vi "WordWrapping.vi"(1 "FormattedMultiLineStringIn":string="123<B>ABCD</B>456\nAAA<B>BBB<I>CCC<U>DDD</U>EEE</I>FFF</B>GGG\n<I>QWERTY</I>\n<U>D<B>123</B>D</U>E", 3 "Font":T3={"Font Name:"="Arial", "Size"=14, "Strikeout?"=FALSE, "Italic?"=FALSE, "Underline?"=FALSE, "Outline?"=FALSE, "Shadow?"=FALSE, "Bold?"=FALSE}, 5 "error in (no error)":errorcluster, 8 "TargetBounds(IgnoreIfZero)":T2 {"height" format="%.2f"; "width" format="%.2f"; "y" format="%.2f"; "x" format="%.2f"}) -> (15 "Width":i16, 16 "Height":i16, 17 "StringWrapped":bool, 18 "WrappedFormattedMultiLineStringOut":string="123<B>ABCD</B>456\nAAA<B>BBB<I>CCC<U>DDD</U>EEE</I>FFF</B>GGG\n<I>QWERTY</I>\n<U>D<B>123</B>D</U>E", 19 "error out":errorcluster)   [LabVIEW 2014, in "Graphics.lvclass"]
uses:
  <resource>/Framework/Providers/Open_GDS/UML/Graphics_class/Graphics.lvclass
  <resource>/Framework/Providers/Open_GDS/UML/General/Rectangle/Rectangle Rectangle2D.ctl
panel:
  out "Array":string[](array[string])
  out "StringsOut":string[](array[string])
  out "Formats":T1(array[cluster])
  # "Layout:\nRemove \\r\\n\nSplit in lines-array\nCalc width per char\nGet number of chars to use for line,\nif rest characters, add these to beggining of  lines-array.\nCalc Bound\nAdd \\r\\n where new lines breaks are"
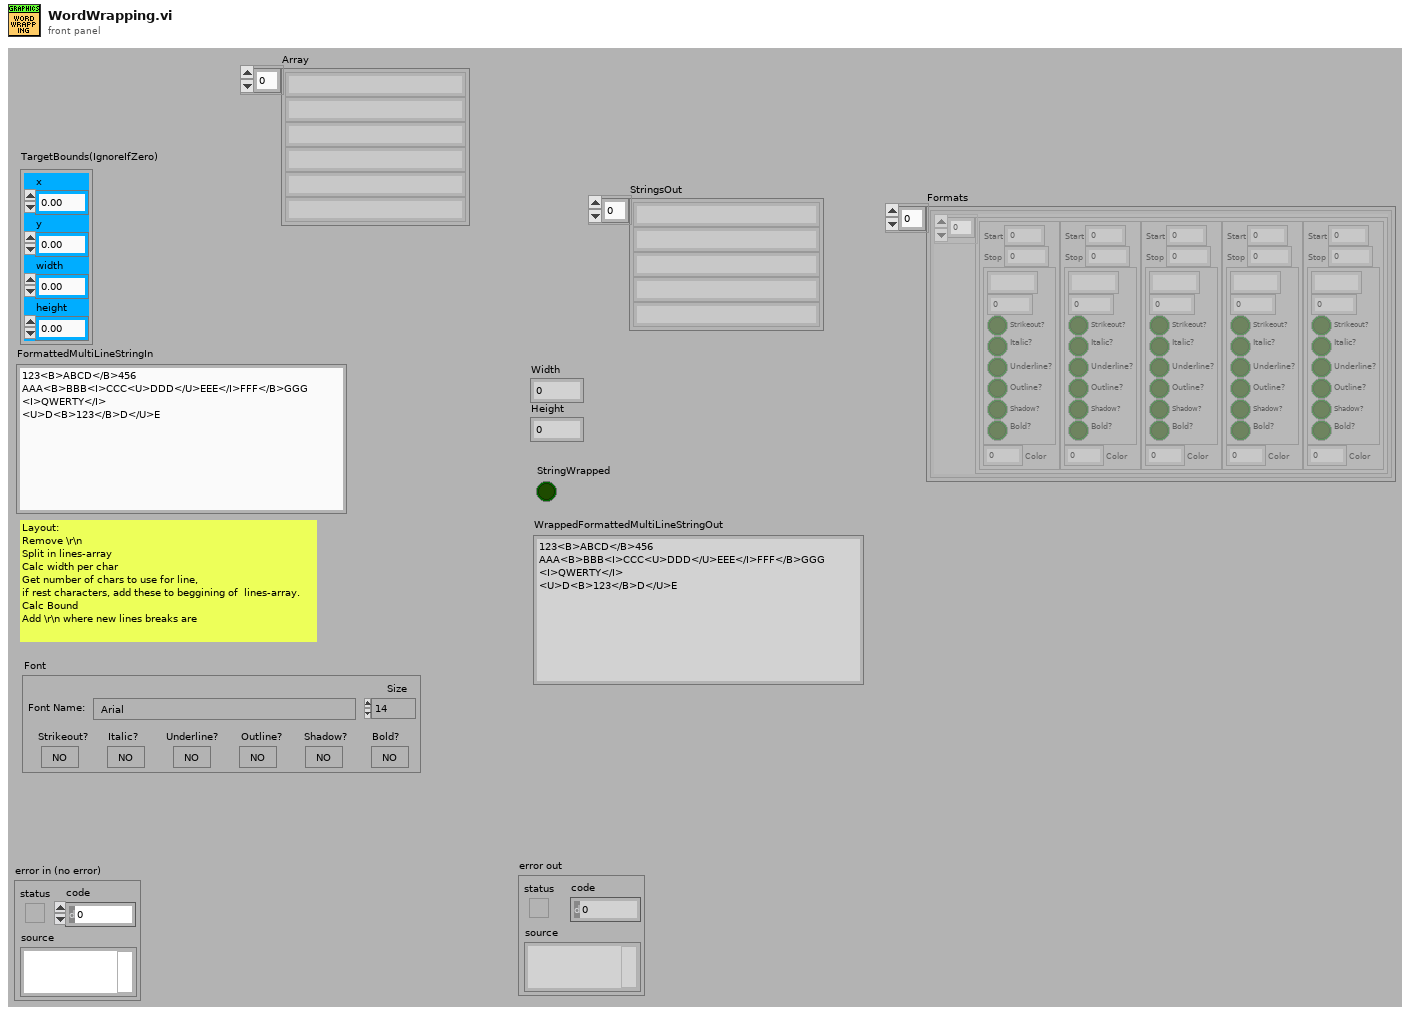
[diagram p1: front panel]
types:
  T1 = cluster{cluster{"Start":i32, "Stop":i32, "Font":cluster{"Font Name:":string, "Size":i16, "Strikeout?":bool, "Italic?":bool, "Underline?":bool, "Outline?":bool, "Shadow?":bool, "Bold?":bool}, "Color":u32}[]}[]
  T2 = typedef "Rectangle Rectangle2D.ctl" = cluster{"x":dbl, "y":dbl, "width":dbl, "height":dbl}
  T3 = cluster{"Font Name:":string, "Size":i16, "Strikeout?":bool, "Italic?":bool, "Underline?":bool, "Outline?":bool, "Shadow?":bool, "Bold?":bool}
  T4 = enum16{"User-specified Font", "Application Font", "System Font", "Dialog Font"}
  T5 = cluster{"Start":i32, "Stop":i32, "Font":cluster{"Font Name:":string, "Size":i16, "Strikeout?":bool, "Italic?":bool, "Underline?":bool, "Outline?":bool, "Shadow?":bool, "Bold?":bool}, "Color":u32}[]
  T6 = cluster{"left":i16, "top":i16, "right":i16, "bottom":i16}
  T7 = cluster{cluster{"Start":i32, "Stop":i32, "Font":cluster{"Font Name:":string, "Size":i16, "Strikeout?":bool, "Italic?":bool, "Underline?":bool, "Outline?":bool, "Shadow?":bool, "Bold?":bool}, "Color":u32}[]}
  T8 = cluster{"Start":i32, "Stop":i32, "Font":cluster{"Font Name:":string, "Size":i16, "Strikeout?":bool, "Italic?":bool, "Underline?":bool, "Outline?":bool, "Shadow?":bool, "Bold?":bool}, "Color":u32}
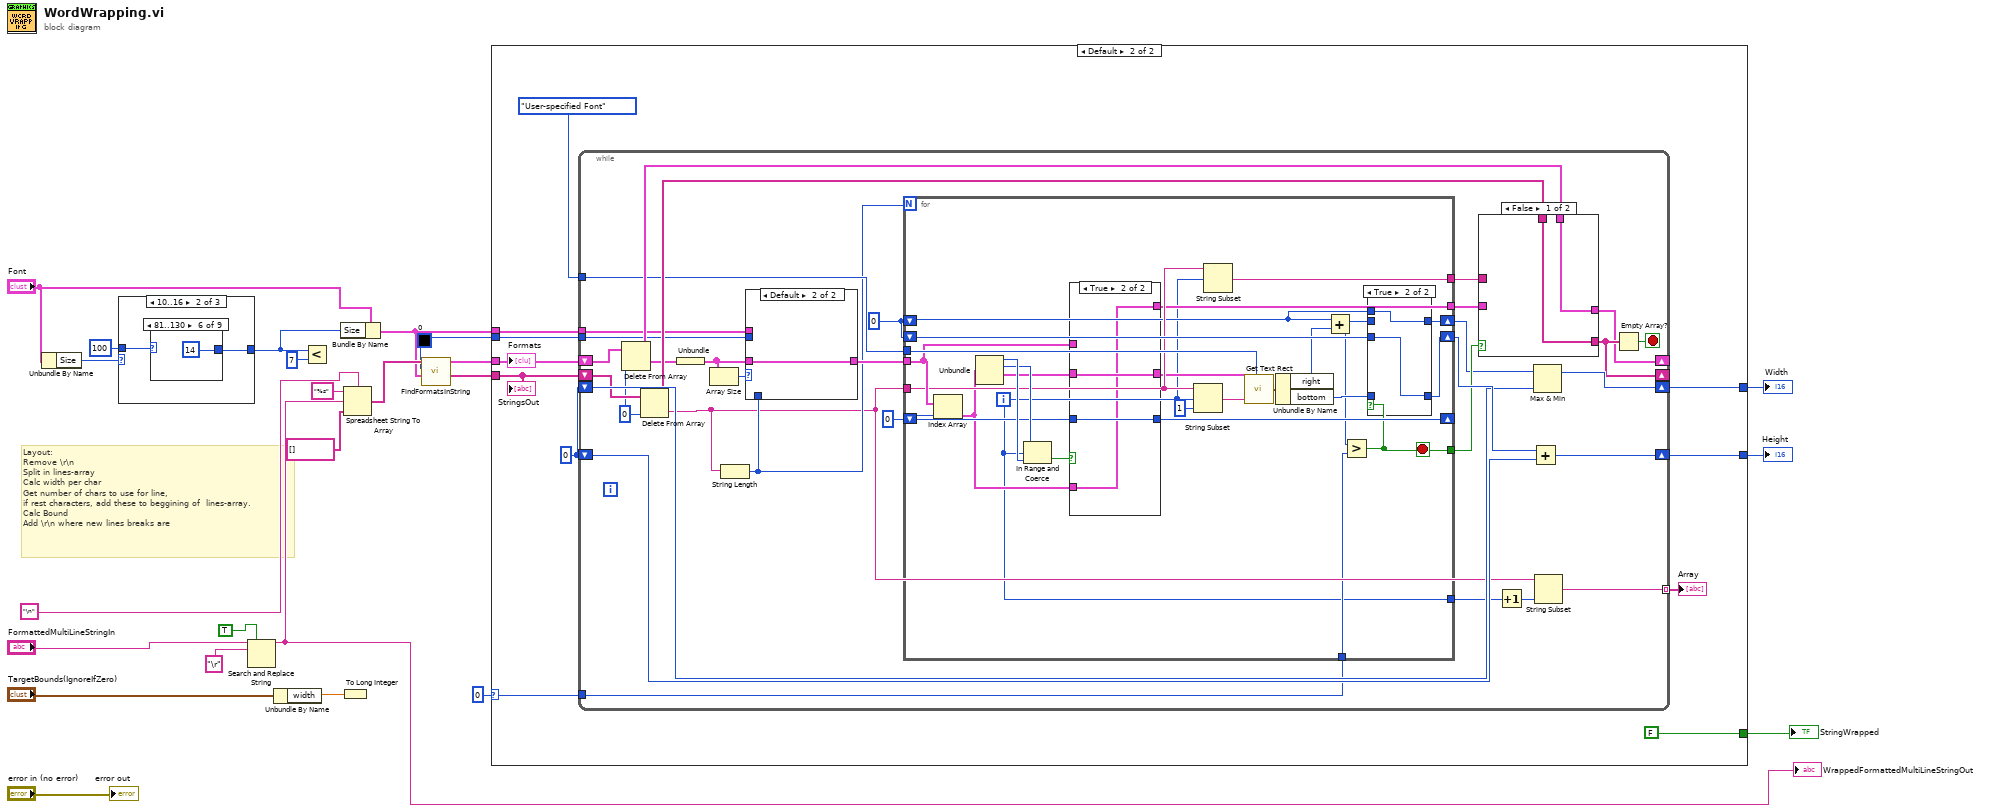
[diagram p0: block diagram]
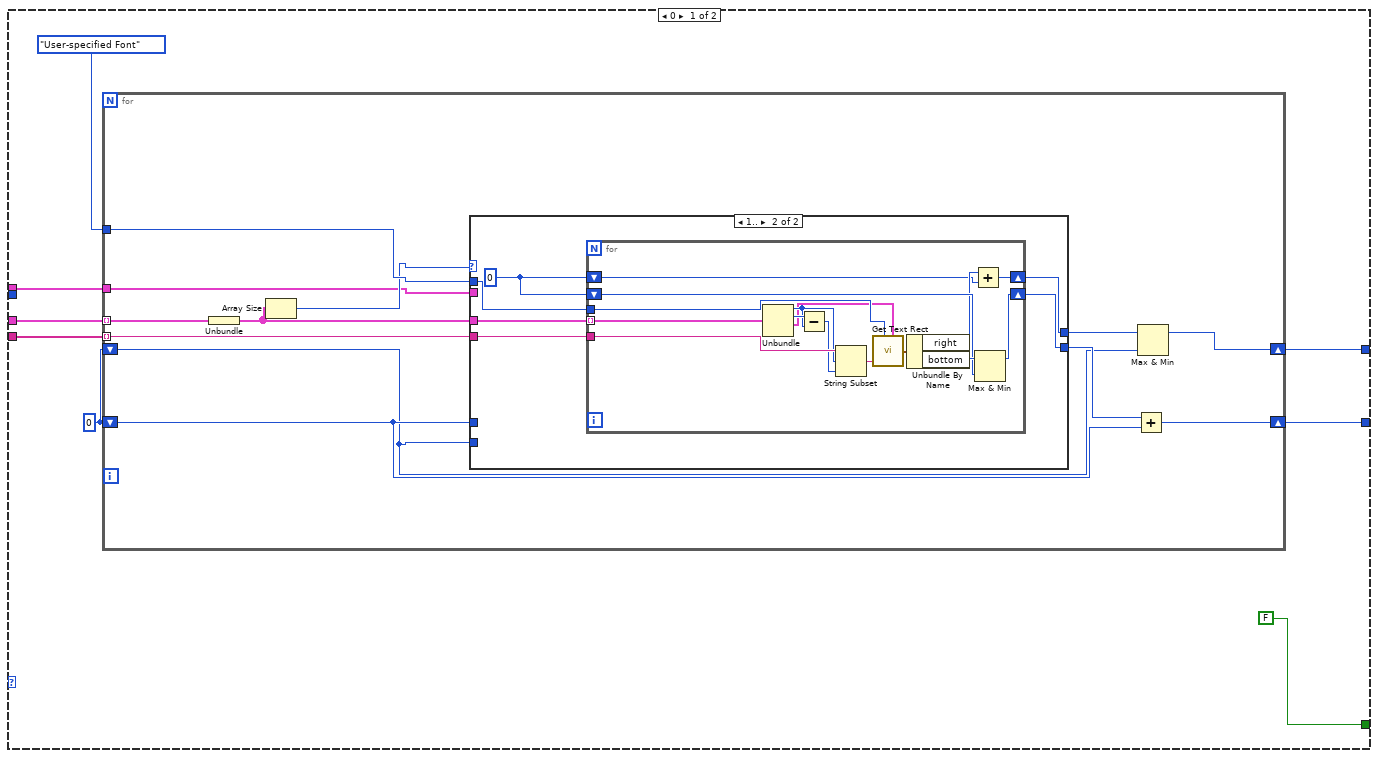
[diagram p2: hidden frame]
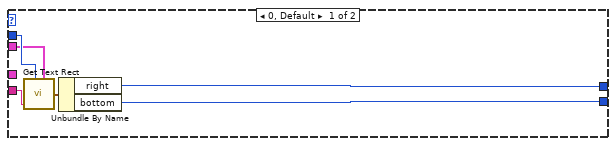
[diagram p3: hidden frame]
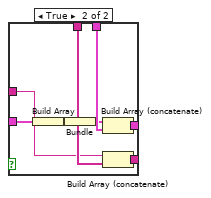
[diagram p4: hidden frame]
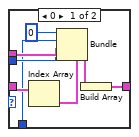
[diagram p5: hidden frame]
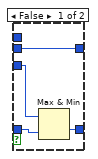
[diagram p6: hidden frame]
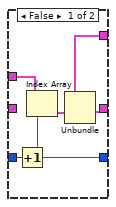
[diagram p7: hidden frame]
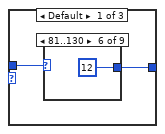
[diagram p8: hidden frame]
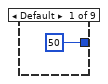
[diagram p9: hidden frame]
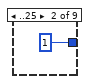
[diagram p10: hidden frame]
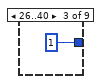
[diagram p11: hidden frame]
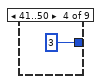
[diagram p12: hidden frame]
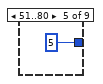
[diagram p13: hidden frame]
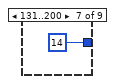
[diagram p14: hidden frame]
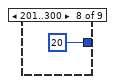
[diagram p15: hidden frame]
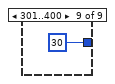
[diagram p16: hidden frame]
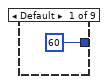
[diagram p17: hidden frame]
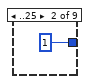
[diagram p18: hidden frame]
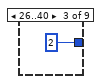
[diagram p19: hidden frame]
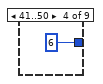
[diagram p20: hidden frame]
diagram:
  w3 = u32 0 ("Color")
  # "Layout:\nRemove \\r\\n\nSplit in lines-array\nCalc width per char\nGet number of chars to use for line,\nif rest characters, add these to beggining of  lines-array.\nCalc Bound\nAdd \\r\\n where new lines breaks are"
  n1 = Unbundle By Name("Font") -> ("Size"=w18:i16)
  n2 = case shown="10..16" w18 {
    tunnel: [w26 w37 w47] -> w17
    tunnel: 100 ("32bit integer") -> [w25 w36 w48]
    frame Default {
      n3 = case shown="81..130" w25 {
        tunnel: [i16 50 ("Size 9") i16 1 ("Size") i16 1 ("Size 2") i16 3 ("Size 3") i16 5 ("Size 4") i16 12 ("Size 5") i16 14 ("Size 6") i16 20 ("Size 7") i16 30 ("Size 8")] -> w26
        frame Default {
        }
        frame ..25 {
        }
        frame 26..40 {
        }
        frame 41..50 {
        }
        frame 51..80 {
        }
        frame 81..130 {
        }
        frame 131..200 {
        }
        frame 201..300 {
        }
        frame 301..400 {
        }
      }
    }
    frame 10..16 {
      n4 = case shown="81..130" w36 {
        tunnel: [i16 60 ("Size 9") i16 1 ("Size") i16 2 ("Size 2") i16 6 ("Size 3") i16 7 ("Size 4") i16 14 ("Size 5") i16 17 ("Size 6") i16 25 ("Size 7") i16 40 ("Size 8")] -> w37
        frame Default {
        }
        frame ..25 {
        }
        frame 26..40 {
        }
        frame 41..50 {
        }
        frame 51..80 {
        }
        frame 81..130 {
        }
        frame 131..200 {
        }
        frame 201..300 {
        }
        frame 301..400 {
        }
      }
    }
    frame 17.. {
      n5 = case shown="201..300" w48 {
        tunnel: [i16 82 ("Size") i16 2 ("Size") i16 5 ("Size") i16 7 ("Size") i16 12 ("Size") i16 18 ("Size") i16 26 ("Size") i16 36 ("Size") i16 55 ("Size")] -> w47
        frame Default {
        }
        frame ..25 {
        }
        frame 26..40 {
        }
        frame 41..50 {
        }
        frame 51..80 {
        }
        frame 81..130 {
        }
        frame 131..200 {
        }
        frame 201..300 {
        }
        frame 301..400 {
        }
      }
    }
  }
  n6 = Search and Replace String(replace all?=TRUE ("replace all? (F)"), input string="FormattedMultiLineStringIn", search string="\r" ("delimiter (Tab)")) -> (result string=w4:string)  [unwired: 5 in, 3 out]
  "WrappedFormattedMultiLineStringOut" <- w4
  n7 = Unbundle By Name("TargetBounds(IgnoreIfZero)") -> ("width"=w5:dbl)
  n8 = Less?(x=w17, y=i16 7) -> ()  [unwired: 1 out]
  n9 = Bundle By Name(cluster="Font", "Size"=w17) -> (w10:T3)
  n10 = To Long Integer(number=w5) -> ()  [unwired: 1 out]
  n11 = Spreadsheet String To Array(delimiter (Tab)="\n", format string="%s", spreadsheet string=w4, array type (2D Dbl)=string[] []) -> (array=w11:string[])
  n12 = call <resource>:"FindFormatsInString.vi"("Font"=w10, "Color"=w3, "StringsIn"=w11) -> ("StringsOut"=w8:string[], "Formats"=w9:T1)  [unwired: 7 in]
  n13 = case shown="Default" 0 {
    selector: 0 -> [_ w106]
    tunnel: [w63 w113] -> w15
    tunnel: [w62 w112] -> w14
    tunnel: w10 -> [w61 w111]
    tunnel: w9 -> [w60 w110]
    tunnel: w8 -> [w59 w109]
    tunnel: [FALSE FALSE] -> w7
    tunnel: w3 -> [_ w107]
    frame 0 {
      w64 = i16 0
      n14 = for {
        tunnel: w60 -> [w77] mode=indexing
        tunnel: w59 -> [w76] mode=indexing
        tunnel: T4."User-specified Font" ("desired font(Application)") -> [w75]
        shift-right: [w74] -> w62
        shift-left: w64 -> [w67]
        shift-right: [w73] -> w63
        shift-left: w64 -> [w66]
        tunnel: w61 -> [w68]
        n15 = Unbundle(w77) -> (w70:T5)
        n16 = Array Size(array=w70) -> (size(s)=w69:i32)
        n17 = case shown="1.." w69 {
          tunnel: w76 -> [w79 w89]
          tunnel: w75 -> [w80 w88]
          tunnel: [w81 w86] -> w72
          tunnel: [w82 w85] -> w71
          tunnel: w70 -> [_ w84]
          tunnel: w68 -> [w78 _]
          tunnel: w67 -> [_ _]
          tunnel: w66 -> [_ _]
          frame 0, Default {
            n18 = call <vilib>:"Get Text Rect.vi"("desired font(Application)"=w80, "text"=w79, "[user-specified font]"=w78) -> ("rect"=w83:T6)  [unwired: 6 in]
            n19 = Unbundle By Name(w83) -> ("right"=w81:i16, "bottom"=w82:i16)
          }
          frame 1.. {
            w87 = i16 0
            n20 = for {
              tunnel: w89 -> [w103]
              tunnel: w84 -> [w104] mode=indexing
              tunnel: w88 -> [w91]
              shift-right: [w94] -> w86
              shift-left: w87 -> [w92]
              shift-right: [w96] -> w85
              shift-left: w87 -> [w97]
              n21 = Unbundle(w104) -> ("Start"=w101:i32, "Stop"=w102:i32, "Font"=w90:T3)  [unwired: 1 out]
              n22 = Subtract(x=w102, y=w101) -> (x-y=w100:i32)
              n23 = String Subset(string=w103, offset (0)=w101, length (rest)=w100) -> (substring=w93:string)
              n24 = call <vilib>:"Get Text Rect.vi"("desired font(Application)"=w91, "text"=w93, "[user-specified font]"=w90) -> ("rect"=w99:T6)  [unwired: 6 in]
              n25 = Unbundle By Name(w99) -> ("right"=w95:i16, "bottom"=w98:i16)
              n26 = Add(x=w95, y=w92) -> (x+y=w94:i16)
              n27 = Max & Min(x=w98, y=w97) -> (max(x,y)=w96:i16)  [unwired: 1 out]
            }
          }
        }
        n28 = Add(x=w71, y=w67) -> (x+y=w74:i16)
        n29 = Max & Min(x=w72, y=w66) -> (max(x,y)=w73:i16)  [unwired: 1 out]
      }
    }
    frame Default {
      w114 = i16 0
      n30 = while {
        tunnel: T4."User-specified Font" ("desired font(Application)") -> [w128]
        shift-right: [w147] -> w112
        shift-left: w114 -> [w144]
        shift-right: [w146] -> w113
        shift-left: w114 -> [w143]
        tunnel: w111 -> [w130]
        shift-right: [w140] -> _
        shift-left: w109 -> [w142]
        shift-right: [w135] -> _
        shift-left: w110 -> [w138]
        tunnel: w107 -> [w129]
        tunnel: w106 -> [w125]
        tunnel: [w116] -> w105 mode=indexing
        stop <- w139 stop-if-true
        w121 = 0 ("index")
        w134 = i16 0
        n31 = Delete From Array(array=w138, index=w121) -> (deleted portion=w137:T7, array with subset deleted=w136:T1)  [unwired: 1 in]
        n32 = Delete From Array(array=w142, index=w121) -> (deleted portion=w117:string, array with subset deleted=w141:string[])  [unwired: 1 in]
        n33 = Unbundle(w137) -> (w132:T5)
        n34 = Array Size(array=w132) -> (size(s)=w133:i32)
        n35 = String Length(string=w117) -> (length=w126:i32)
        n36 = case shown="Default" w133 {
          tunnel: w132 -> [w165 w166]
          tunnel: [w159 w166] -> w131
          tunnel: w130 -> [w162 _]
          tunnel: w129 -> [w161 _]
          tunnel: w126 -> [w158 _]
          frame 0 {
            n37 = Index Array(array=w165) -> (element=w164:T8)  [unwired: 1 in]
            n38 = Bundle(cluster=w164, "Start"=0, "Stop"=w158, "Font"=w162, "Color"=w161) -> (w160:T8)
            n39 = Build Array(w160) -> (w159:T5)
          }
          frame Default {
          }
        }
        n40 = for {
          N: w126 -> [_]
          tunnel: w117 -> [w177]
          tunnel: w131 -> [w179]
          tunnel: w128 -> [w186]
          shift-right: [w169] -> w120
          shift-left: w134 -> [w168]
          shift-right: [w189] -> w145
          shift-left: w134 -> [w190]
          shift-right: [w180] -> _
          shift-left: i16 0 -> [w181]
          tunnel: w125 -> [w178]
          tunnel: [w171] -> w124
          tunnel: [w176] -> w123
          tunnel: [w174] -> w122
          tunnel: [w167] -> w119
          i -> [w167]
          stop <- w171 stop-if-true
          n41 = Index Array(array=w179, index=w181) -> (element=w173:T8)
          n42 = Unbundle(w173) -> ("Start"=w185:i32, "Stop"=w184:i32, "Font"=w182:T3)  [unwired: 1 out]
          n43 = In Range and Coerce(upper limit=w184, x=w167, lower limit=w185) -> (In Range?=w183:bool)  [unwired: 1 out]
          n44 = case shown="True" w183 {
            tunnel: w182 -> [_ w205]
            tunnel: w181 -> [w203 w206]
            tunnel: [w201 w206] -> w180
            tunnel: [w200 w205] -> w175
            tunnel: w179 -> [w202 _]
            tunnel: [w199 w204] -> w174
            tunnel: w173 -> [_ w204]
            frame False {
              n45 = Increment(x=w203) -> (x+1=w201:i16)
              n46 = Index Array(array=w202, index=w201) -> (element=w199:T8)
              n47 = Unbundle(w199) -> ("Font"=w200:T3)  [unwired: 3 out]
            }
            frame True {
            }
          }
          n48 = String Subset(string=w177, offset (0)=w167, length (rest)=1 ("length (rest)")) -> (substring=w188:string)
          n49 = String Subset(string=w177, offset (0)=w167) -> (substring=w176:string)  [unwired: 1 in]
          n50 = call <vilib>:"Get Text Rect.vi"("desired font(Application)"=w186, "text"=w188, "[user-specified font]"=w175) -> ("rect"=w192:T6)  [unwired: 6 in]
          n51 = Unbundle By Name(w192) -> ("right"=w172:i16, "bottom"=w191:i16)
          n52 = Add(x=w168, y=w172) -> (x+y=w170:i16)
          n53 = Greater?(x=w170, y=w178) -> (0:w171:bool)
          n54 = case shown="True" w171 {
            tunnel: w191 -> [w196 _]
            tunnel: w190 -> [w195 w198]
            tunnel: [w194 w198] -> w189
            tunnel: w170 -> [w193 _]
            tunnel: [w193 w197] -> w169
            tunnel: w168 -> [_ w197]
            frame False {
              n55 = Max & Min(x=w195, y=w196) -> (max(x,y)=w194:i16)  [unwired: 1 out]
            }
            frame True {
            }
          }
        }
        n56 = case shown="False" w124 {
          tunnel: w141 -> [w148 w157]
          tunnel: [w148 w156] -> w140
          tunnel: w136 -> [w149 w155]
          tunnel: [w149 w154] -> w135
          tunnel: w123 -> [_ w153]
          tunnel: w122 -> [_ w152]
          frame False {
          }
          frame True {
            n57 = Build Array(w152) -> (w150:T5)
            n58 = Bundle(w150) -> (w151:T7)  [unwired: 1 in]
            n59 = Build Array (concatenate)(w151, w155) -> (w154:T1)
            n60 = Build Array (concatenate)(w153, w157) -> (w156:string[])
          }
        }
        n61 = Increment(x=w119) -> (x+1=w118:i32)
        n62 = Add(x=w145, y=w144) -> (x+y=w147:i16)
        n63 = Max & Min(x=w120, y=w143) -> (max(x,y)=w146:i16)  [unwired: 1 out]
        n64 = String Subset(string=w117, length (rest)=w118) -> (substring=w116:string)  [unwired: 1 in]
        n65 = Empty Array?(array=w140) -> (empty?=w139:bool)
      }
      "Array" <- w105
      "Formats" <- w110
      "StringsOut" <- w109
    }
  }
  "Width" <- w15
  "Height" <- w14
  "StringWrapped" <- w7
  "error out" <- "error in (no error)"
